vi "XML Parse DBL.vi"(3 "Attribut Name":string, 7 "XML Response":string) -> (0 "Wert (DBL)":dbl, 2 "XML Response gekürzt":string)   [LabVIEW 2020, in "FT-IR.lvlib" / "TOOLweb Interface.lvlib" / "TOOLweb Interface Hilfs-VIs.lvlib"]
doc: "Sucht in dem XML-Poll-Response-String \"XML-Response\" den Eintrag mit dem Elementnamen \"Attribut Name\" und liefert dessen Wert in \"Wert (DBL)\". \n\nDer Eintrag wird dann entfernt, damit eine weiteres Parser-VI am Ausgang \"XML Response gekürzt\" nicht wieder den ganzen String durchsuchen muss."
uses:
  TOOLweb Interface Hilfs-VIs.lvlib
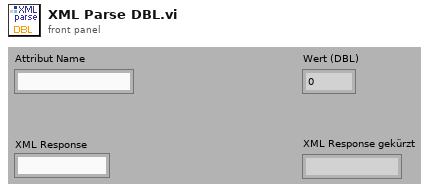
[diagram p1: front panel]
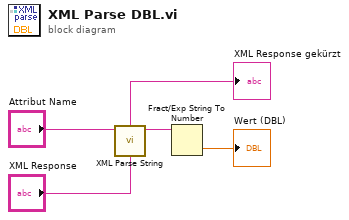
[diagram p0: block diagram]
diagram:
  n1 = call "XML Parse String.vi"("Attribut Name"="Attribut Name", "XML Response"="XML Response") -> ("Wert-String"=w2:string, "XML Response gekürzt"=→"XML Response gekürzt":string)  [unwired: 6 out]
  n2 = Fract/Exp String To Number(string=w2) -> (number=→"Wert (DBL)":dbl)  [unwired: 4 out]
